vi "Conditional Clear Error.vi"(7 "String Array":string[](array[string]), 8 "error in (no error)":errorcluster, 11 "Search String":string) -> (0 "error out":errorcluster, 2 "Error Cleared?":bool)   [LabVIEW 2016, in "Stream Error.lvlib"]
doc: "--\nCopyright © 2017 Composed SystemsI All rights reserved.\n\nAuthor: Jon McBee <jon.mcbee@composed.io>\n\nThis library is provided \"AS IS\" ,WITHOUT WARRANTIES OR\nCONDITIONS OF ANY KIND, either express or implied.\n\nComposed Systems -- composed.io\n\nStream 0.0.1.1\nJon McBee - Composed Systems\nCopyright (c) 2017, Composed Systems"
uses:
  <userlib>/Composed Systems/Stream/Error/Stream Error.lvlib
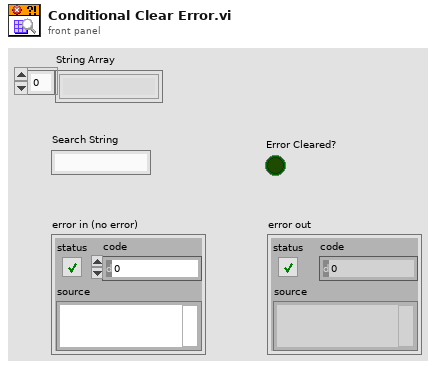
[diagram p1: front panel]
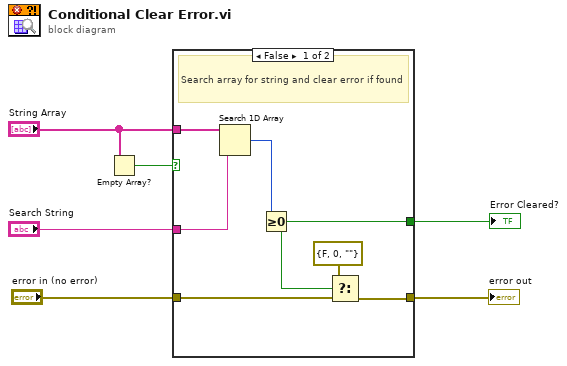
[diagram p0: block diagram]
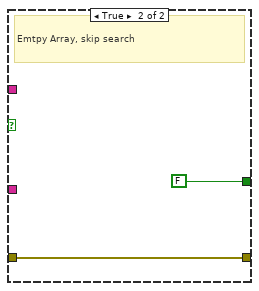
[diagram p2: hidden frame]
diagram:
  n1 = Empty Array?(array="String Array") -> (empty?=w6:bool)
  n2 = case shown="False" w6 {
    tunnel: "String Array" -> [w13 _]
    tunnel: "Search String" -> [w12 _]
    tunnel: [w8 w15] -> w3
    tunnel: "error in (no error)" -> [w10 w15]
    tunnel: [w9 FALSE] -> w1
    frame False {
      # "Search array for string and clear error if found"
      n3 = Search 1D Array(1D array=w13, element=w12) -> (index of element=w11:i32)  [unwired: 1 in]
      n4 = Greater Or Equal To 0?(x=w11) -> (x >= 0?=w9:bool)
      n5 = Select(t=errorcluster {"status"=FALSE, "code"=0, "source"=""}, s=w9, f=w10) -> (s? t:f=w8:errorcluster)
    }
    frame True {
      # "Emtpy Array, skip search"
    }
  }
  "Error Cleared?" <- w1
  "error out" <- w3
